vi "File Viewer.vi"() -> ()   [LabVIEW 2015]
uses:
  <vilib>/FileIngestion/FileIngestion.lvlib
  <vilib>/FileIngestion/AvailableFileEvent.lvclass
panel:
  in  "stop":bool
  out "Number of files":i32
  out "Files":string[][](table)
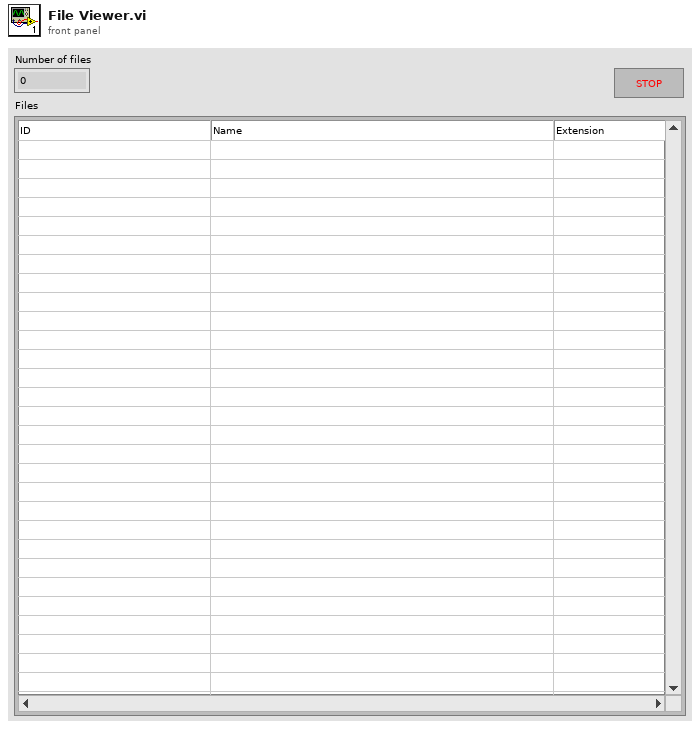
[diagram p1: front panel]
types:
  T1 = cluster{"id":string, "properties":cluster{"key":string, "value":string}[]}[]
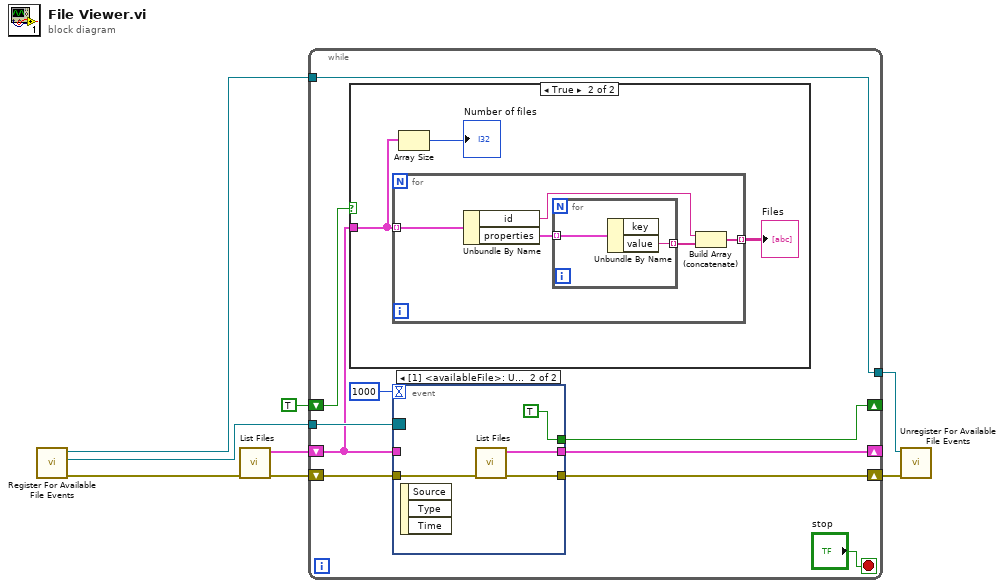
[diagram p0: block diagram]
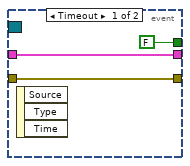
[diagram p3: hidden frame]
diagram:
  n1 = call <vilib>:"Register For Available File Events.vi"() -> ("error out"=w4:errorcluster, "event registration refnum"=w8:refnum<event-registration>, "output cluster"=w6:refnum<class "AvailableFileEvent.lvclass">)  [unwired: 9 in]
  n2 = call <vilib>:"List Files.vi"("error in"=w4) -> ("error out"=w3:errorcluster, "available files"=w2:T1)  [unwired: 7 in]
  n3 = while {
    tunnel: w8 -> [w17]
    tunnel: w6 -> [w14]
    tunnel: [w14] -> w5
    shift-right: [w11] -> _
    shift-left: w2 -> [w12]
    shift-right: [w10] -> _
    shift-left: TRUE -> [w9]
    shift-right: [w15] -> w7
    shift-left: w3 -> [w16]
    stop <- "stop" stop-if-true
    n4 = case shown="True" w9 {
      tunnel: w12 -> [_ w19]
      frame False {
      }
      frame True {
        n5 = for {
          tunnel: w19 -> [w26] mode=indexing
          tunnel: [w22] -> w21 mode=indexing
          n6 = Unbundle By Name(w26) -> ("id"=w24:string, "properties"=w25:cluster{"key":string, "value":string}[])
          n7 = for {
            tunnel: w25 -> [w28] mode=indexing
            tunnel: [w27] -> w23 mode=indexing
            n8 = Unbundle By Name(w28) -> ("value"=w27:string)  [unwired: 1 out]
          }
          n9 = Build Array (concatenate)(w24, w23) -> (w22:string[])
        }
        "Files" <- w21
        n10 = Array Size(array=w19) -> (size(s)=→"Number of files":i32)
      }
    }
    n11 = event shown="[1] <availableFile>: User Event" {
      selector: w17 -> [_ _]
      dyn-events: _ -> [_ _]
      timeout: u32 1000 ("millisecond multiple") -> [_ _]
      tunnel: [w31 w35] -> w11
      tunnel: w16 -> [w30 w33]
      tunnel: [w30 w34] -> w15
      tunnel: w12 -> [w31 _]
      tunnel: [FALSE TRUE] -> w10
      event Timeout {
        n12 = event-data() -> ()  [unwired: 1 in, 3 out]
      }
      event User Event {
        n13 = event-data() -> ()  [unwired: 1 in, 3 out]
        n14 = call <vilib>:"List Files.vi"("error in"=w33) -> ("error out"=w34:errorcluster, "available files"=w35:T1)  [unwired: 7 in]
      }
    }
  }
  n15 = call <vilib>:"Unregister For Available File Events.vi"("error in"=w7, "FileIngestion.lvlib:AvailableFileEvent.lvclass"=w5) -> ()  [unwired: 9 in, 1 out]
